vi "Create Client from Template.vi"(8 "error in (no error)":errorcluster, 9 "Generated Server Name":string="Generated Server", 10 "Target Project Path":path, 11 "Application ref in":refnum<vi>) -> (0 "error out":errorcluster, 1 "Already exists ?":bool, 2 "Server class out":refnum<vi>, 3 "Server library out":refnum<vi>)   [LabVIEW 2019, in "gRPC Scripting Tools.lvlib"]
uses:
  gRPC Scripting Tools.lvlib
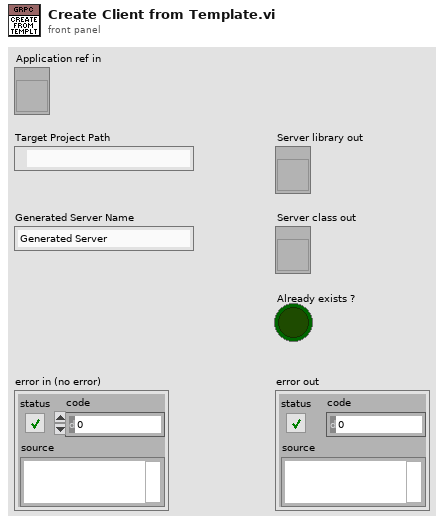
[diagram p1: front panel]
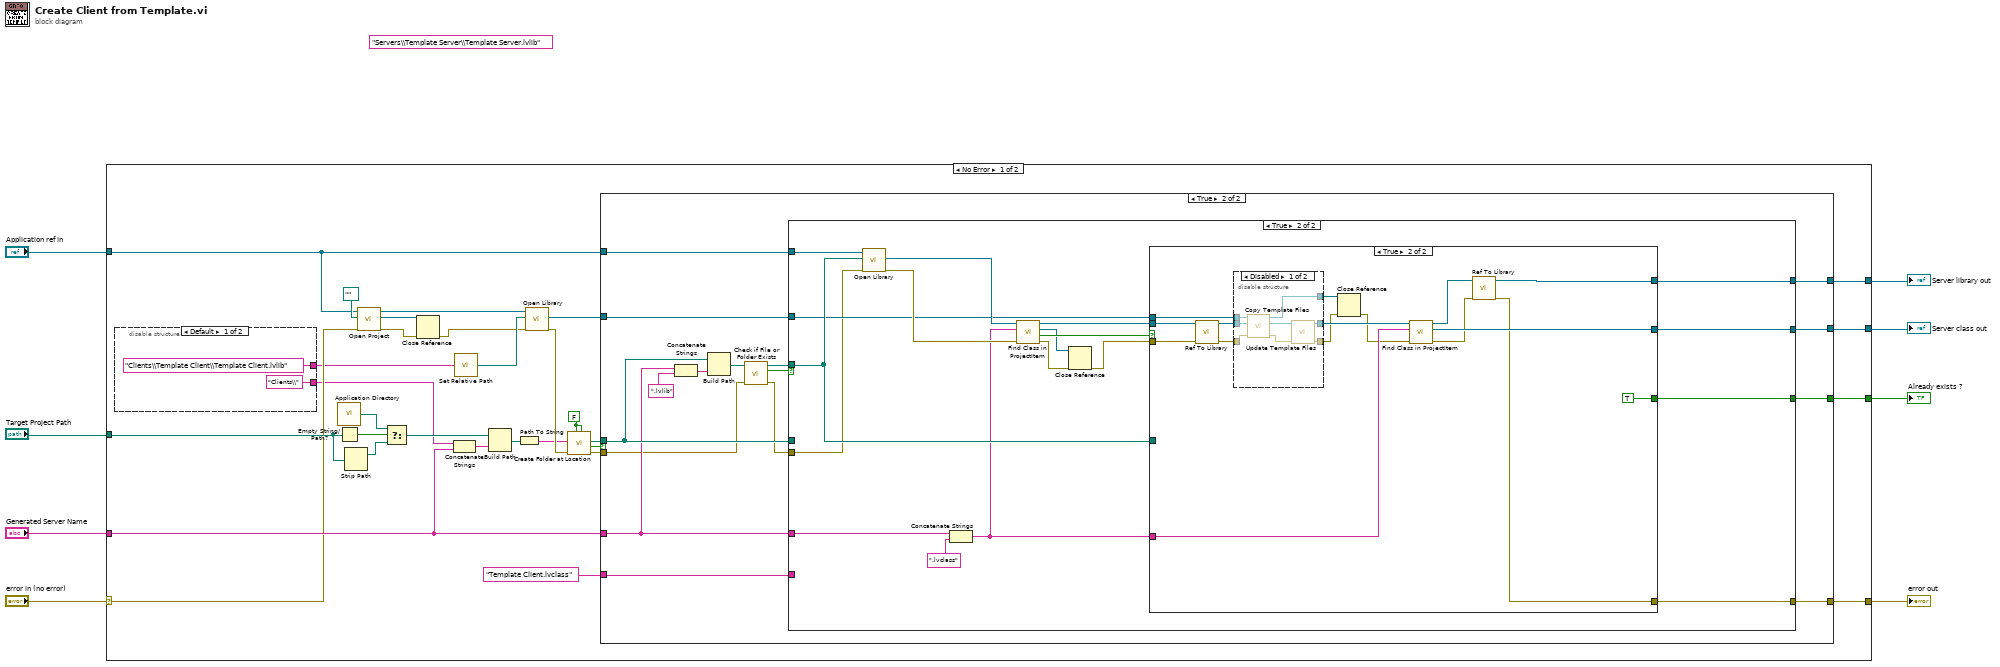
[diagram p0: block diagram]
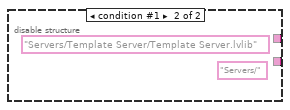
[diagram p2: hidden frame]
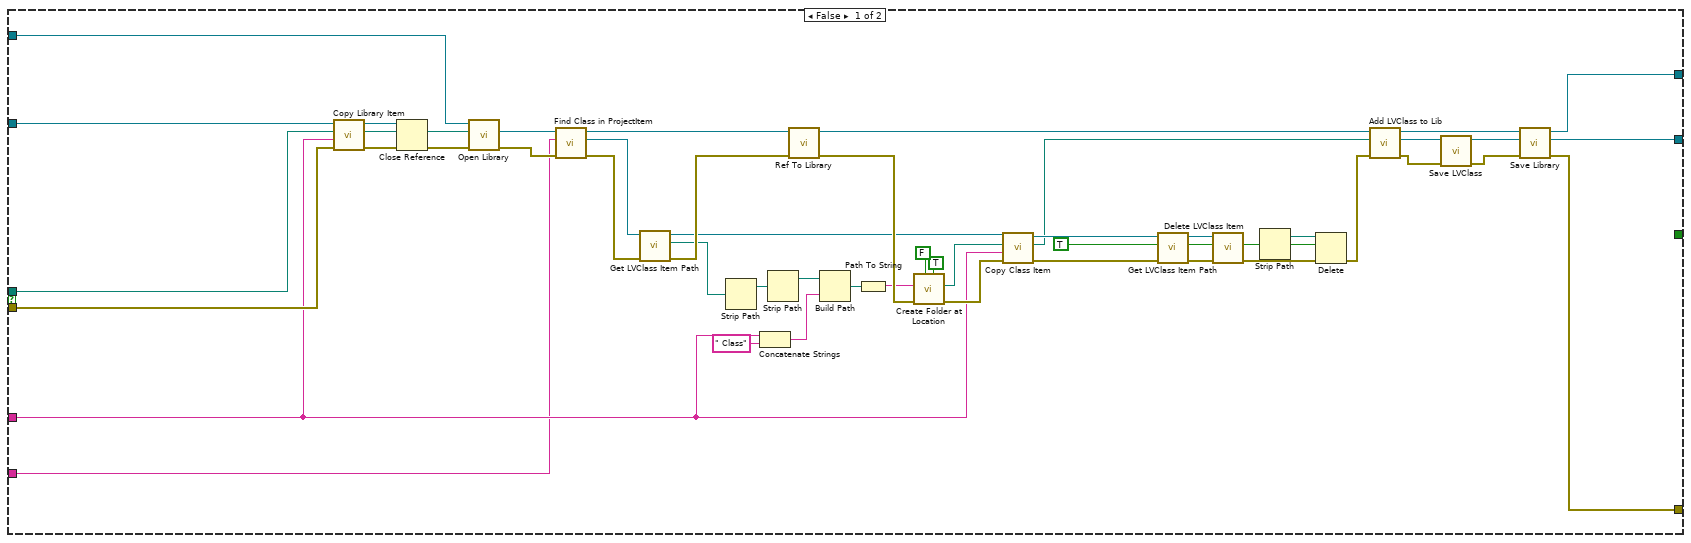
[diagram p3: hidden frame]
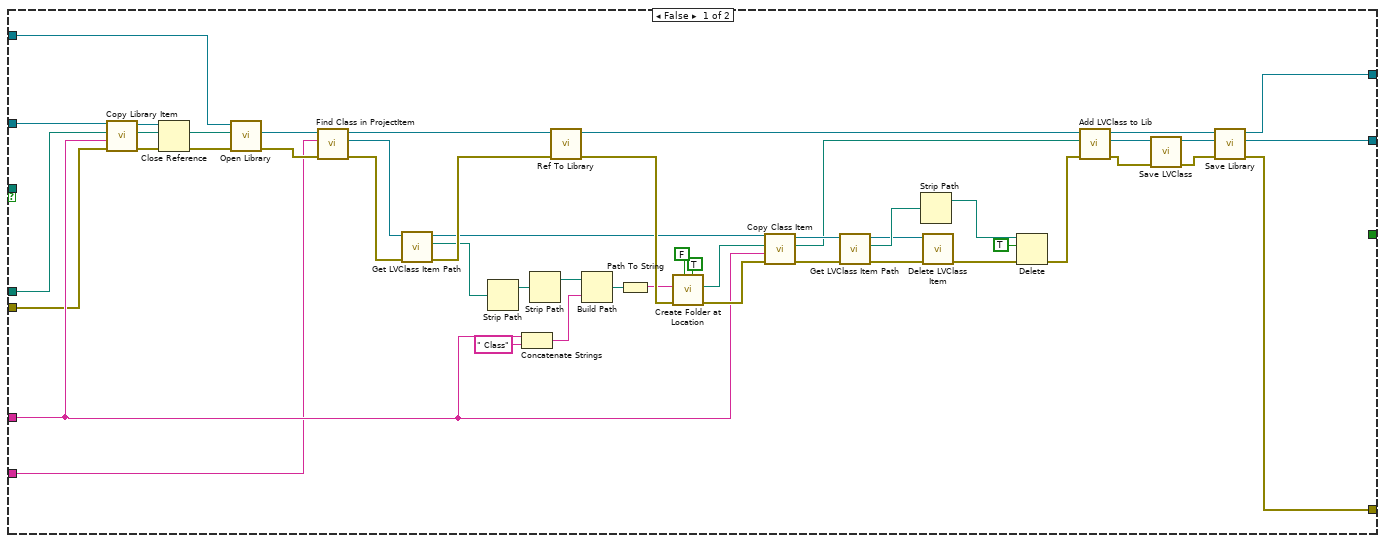
[diagram p4: hidden frame]
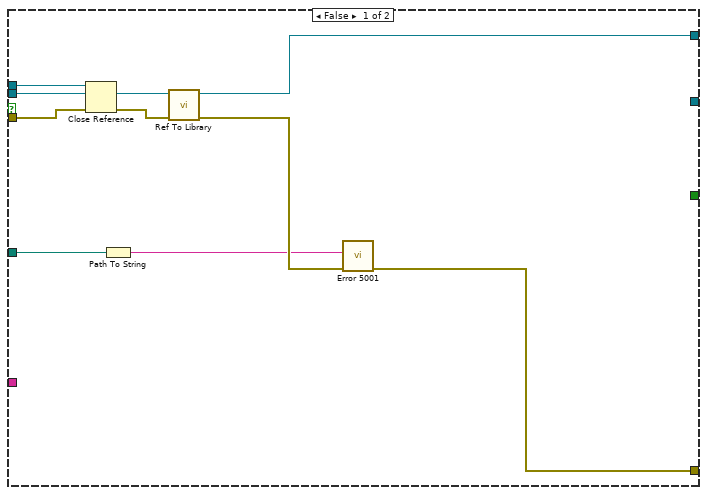
[diagram p5: hidden frame]
diagram:
  (unwired) "Servers\\Template Server\\Template Server.lvlib" ("Application Relative Path")
  n1 = case shown="No Error" "error in (no error)" {
    selector: "error in (no error)" -> [w14 w205]
    tunnel: [w38 w205] -> w8
    tunnel: [w37 _] -> w7
    tunnel: [w36 _] -> w6
    tunnel: "Target Project Path" -> [w17 _]
    tunnel: "Generated Server Name" -> [w16 _]
    tunnel: "Application ref in" -> [w15 _]
    tunnel: [w12 _] -> w1
    frame No Error {
      w29 = FALSE ("Use Relative")
      n2 = disable-structure shown="Default" {
        disable-tunnel: ["Clients\\Template Client\\Template Client.lvlib" ("Application Relative Path") _] -> w11
        disable-tunnel: ["Clients\\" ("Path") _] -> w10
        frame condition #0 (active) {
        }
        frame condition #1 {
          (unwired) "Servers/" ("Path")
          (unwired) "Servers/Template Server/Template Server.lvlib" ("Application Relative Path")
        }
      }
      n3 = call <vilib>:"Application Directory.vi"() -> ("Application Directory"=w18:path)
      n4 = Empty String/Path?(string/path=w17) -> (empty?=w21:bool)
      n5 = Strip Path(path=w17) -> (stripped path=w20:path)  [unwired: 1 out]
      n6 = call "Open Project.vi"("error in (no error)"=w14, "Project Path in"=path "", "Application reference"=w15) -> ("error out"=w24:errorcluster, "Project out"=w25:refnum<vi>, "Application out"=w32:refnum<vi>)  [unwired: 6 in]
      n7 = Select(t=w18, s=w21, f=w20) -> (s? t:f=w19:path)
      n8 = Close Reference(reference=w25, error in (no error)=w24) -> (error out=w23:errorcluster)
      n9 = Concatenate Strings(w10, w16) -> (w28:string)
      n10 = call "Set Relative Path.vi"("Application Relative Path"=w11) -> ("Full Path"=w33:path)
      n11 = Build Path(base path=w19, name or relative path=w28) -> (appended path=w27:path)
      n12 = Path To String(path=w27) -> (string=w26:string)
      n13 = call "Open Library.vi"("error in (no error)"=w23, "Full Path"=w33, "Application in"=w32) -> ("error out"=w34:errorcluster, "Library out"=w30:refnum<vi>)  [unwired: 6 in, 1 out]
      n14 = call "Create Folder at Location.vi"("Override existing (F)"=w29, "Use Relative (F)"=w29, "Error In"=w34, "Path"=w26) -> ("Error Out"=w35:errorcluster, "Already Exists ?"=w13:bool, "Full path out"=w31:path)  [unwired: 5 in]
      n15 = case shown="True" w13 {
        tunnel: [w87 w93] -> w38
        tunnel: [w86 w98] -> w37
        tunnel: [w85 w99] -> w36
        tunnel: w35 -> [w50 w90]
        tunnel: w31 -> [w49 w95]
        tunnel: w30 -> [w48 w96]
        tunnel: w16 -> [w43 w94]
        tunnel: w15 -> [w42 w97]
        tunnel: [_ w92] -> w12
        tunnel: "Template Client.lvclass" ("Class Name") -> [w41 w88]
        frame False {
          n16 = call "Copy Library Item.vi"("error in (no error)"=w50, "Copy Name"=w43, "Copy location"=w49, "Library in"=w48) -> ("error out"=w70:errorcluster, "New Lib Path"=w47:path, "Library out"=w69:refnum<vi>)  [unwired: 5 in]
          n17 = Close Reference(reference=w69, error in (no error)=w70) -> (error out=w46:errorcluster)
          n18 = call "Open Library.vi"("error in (no error)"=w46, "Full Path"=w47, "Application in"=w42) -> ("error out"=w44:errorcluster, "Library out"=w45:refnum<vi>)  [unwired: 6 in, 1 out]
          n19 = call "Find Class in ProjectItem.vi"("error in (no error)"=w44, "Class Name"=w41, "ProjectItem in"=w45) -> ("error out"=w52:errorcluster, "LVClass out"=w51:refnum<vi>, "ProjectItem out"=w64:refnum<vi>)  [unwired: 5 in, 1 out]
          n20 = call "Get LVClass Item Path.vi"("error in (no error)"=w52, "LVClassLibrary in"=w51) -> ("error out"=w66:errorcluster, "Path"=w53:path, "LVClassLibrary out"=w54:refnum<vi>)  [unwired: 7 in]
          n21 = Strip Path(path=w53) -> (stripped path=w62:path)  [unwired: 1 out]
          n22 = Concatenate Strings(w43, " Class" ("string")) -> (w57:string)
          n23 = Strip Path(path=w62) -> (stripped path=w63:path)  [unwired: 1 out]
          n24 = call "Ref To Library.vi"("error in (no error)"=w66, "ProjectItem in"=w64) -> ("error out"=w67:errorcluster, "Library out"=w80:refnum<vi>)  [unwired: 8 in]
          n25 = Build Path(base path=w63, name or relative path=w57) -> (appended path=w58:path)
          n26 = Path To String(path=w58) -> (string=w59:string)
          n27 = call "Create Folder at Location.vi"("Override existing (F)"=TRUE, "Use Relative (F)"=FALSE ("Use Relative"), "Error In"=w67, "Path"=w59) -> ("Error Out"=w68:errorcluster, "Full path out"=w61:path)  [unwired: 5 in, 1 out]
          n28 = call "Copy Class Item.vi"("error in (no error)"=w68, "New Name"=w43, "Full path in"=w61, "LVClassLibrary in"=w54) -> ("error out"=w72:errorcluster, "New Class Path out"=w65:path, "LVClassLibrary out"=w71:refnum<vi>)  [unwired: 5 in]
          n29 = call "Get LVClass Item Path.vi"("error in (no error)"=w72, "LVClassLibrary in"=w71) -> ("error out"=w74:errorcluster, "Path"=w75:path, "LVClassLibrary out"=w73:refnum<vi>)  [unwired: 7 in]
          n30 = call "Delete LVClass Item.vi"("error in (no error)"=w74, "LVClassLibrary in"=w73) -> ("error out"=w77:errorcluster)  [unwired: 9 in]
          n31 = Strip Path(path=w75) -> (stripped path=w76:path)  [unwired: 1 out]
          n32 = Delete(path (use dialog)=w76, entire hierarchy (F)=TRUE, error in=w77) -> (error out=w78:errorcluster)  [unwired: 2 in, 2 out]
          n33 = call "Add LVClass to Lib.vi"("error in (no error)"=w78, "LVClass Path in"=w65, "Library in"=w80) -> ("error out"=w83:errorcluster, "LVClassLibrary out"=w82:refnum<vi>, "Library out"=w81:refnum<vi>)  [unwired: 6 in]
          n34 = call "Save LVClass.vi"("error in (no error)"=w83, "LVClassLibrary in"=w82) -> ("error out"=w84:errorcluster, "LVClassLibrary out"=w86:refnum<vi>)  [unwired: 8 in]
          n35 = call "Save Library.vi"("error in (no error)"=w84, "Library in"=w81) -> ("error out"=w87:errorcluster, "Library out"=w85:refnum<vi>)  [unwired: 8 in]
        }
        frame True {
          n36 = Concatenate Strings(w94, ".lvlib" ("string")) -> (w102:string)
          n37 = Build Path(base path=w95, name or relative path=w102) -> (appended path=w101:path)
          n38 = call <vilib>:"Check if File or Folder Exists.vi"("error in (no error)"=w90, "path"=w101) -> ("error out"=w89:errorcluster, "file or folder exists?"=w100:bool, "dup path"=w91:path)  [unwired: 7 in]
          n39 = case shown="True" w100 {
            tunnel: [w112 w162] -> w99
            tunnel: [w111 w151] -> w98
            tunnel: w97 -> [w110 w168]
            tunnel: w96 -> [w109 w157]
            tunnel: w95 -> [w108 _]
            tunnel: w94 -> [w107 w166]
            tunnel: w89 -> [w106 w156]
            tunnel: [w105 w161] -> w93
            tunnel: [_ w159] -> w92
            tunnel: w91 -> [_ w158]
            tunnel: w88 -> [w104 _]
            frame False {
              n40 = call "Copy Library Item.vi"("error in (no error)"=w106, "Copy Name"=w107, "Copy location"=w108, "Library in"=w109) -> ("error out"=w136:errorcluster, "New Lib Path"=w116:path, "Library out"=w135:refnum<vi>)  [unwired: 5 in]
              n41 = Close Reference(reference=w135, error in (no error)=w136) -> (error out=w115:errorcluster)
              n42 = call "Open Library.vi"("error in (no error)"=w115, "Full Path"=w116, "Application in"=w110) -> ("error out"=w113:errorcluster, "Library out"=w114:refnum<vi>)  [unwired: 6 in, 1 out]
              n43 = call "Find Class in ProjectItem.vi"("error in (no error)"=w113, "Class Name"=w104, "ProjectItem in"=w114) -> ("error out"=w118:errorcluster, "LVClass out"=w117:refnum<vi>, "ProjectItem out"=w130:refnum<vi>)  [unwired: 5 in, 1 out]
              n44 = call "Get LVClass Item Path.vi"("error in (no error)"=w118, "LVClassLibrary in"=w117) -> ("error out"=w132:errorcluster, "Path"=w119:path, "LVClassLibrary out"=w120:refnum<vi>)  [unwired: 7 in]
              n45 = Strip Path(path=w119) -> (stripped path=w128:path)  [unwired: 1 out]
              n46 = Concatenate Strings(w107, " Class" ("string")) -> (w123:string)
              n47 = Strip Path(path=w128) -> (stripped path=w129:path)  [unwired: 1 out]
              n48 = call "Ref To Library.vi"("error in (no error)"=w132, "ProjectItem in"=w130) -> ("error out"=w133:errorcluster, "Library out"=w146:refnum<vi>)  [unwired: 8 in]
              n49 = Build Path(base path=w129, name or relative path=w123) -> (appended path=w124:path)
              n50 = Path To String(path=w124) -> (string=w125:string)
              n51 = call "Create Folder at Location.vi"("Override existing (F)"=TRUE, "Use Relative (F)"=FALSE ("Use Relative"), "Error In"=w133, "Path"=w125) -> ("Error Out"=w134:errorcluster, "Full path out"=w127:path)  [unwired: 5 in, 1 out]
              n52 = call "Copy Class Item.vi"("error in (no error)"=w134, "New Name"=w107, "Full path in"=w127, "LVClassLibrary in"=w120) -> ("error out"=w138:errorcluster, "New Class Path out"=w131:path, "LVClassLibrary out"=w137:refnum<vi>)  [unwired: 5 in]
              n53 = call "Get LVClass Item Path.vi"("error in (no error)"=w138, "LVClassLibrary in"=w137) -> ("error out"=w140:errorcluster, "Path"=w141:path, "LVClassLibrary out"=w139:refnum<vi>)  [unwired: 7 in]
              n54 = Strip Path(path=w141) -> (stripped path=w142:path)  [unwired: 1 out]
              n55 = call "Delete LVClass Item.vi"("error in (no error)"=w140, "LVClassLibrary in"=w139) -> ("error out"=w143:errorcluster)  [unwired: 9 in]
              n56 = Delete(path (use dialog)=w142, entire hierarchy (F)=TRUE, error in=w143) -> (error out=w144:errorcluster)  [unwired: 2 in, 2 out]
              n57 = call "Add LVClass to Lib.vi"("error in (no error)"=w144, "LVClass Path in"=w131, "Library in"=w146) -> ("error out"=w149:errorcluster, "LVClassLibrary out"=w148:refnum<vi>, "Library out"=w147:refnum<vi>)  [unwired: 6 in]
              n58 = call "Save LVClass.vi"("error in (no error)"=w149, "LVClassLibrary in"=w148) -> ("error out"=w150:errorcluster, "LVClassLibrary out"=w111:refnum<vi>)  [unwired: 8 in]
              n59 = call "Save Library.vi"("error in (no error)"=w150, "Library in"=w147) -> ("error out"=w105:errorcluster, "Library out"=w112:refnum<vi>)  [unwired: 8 in]
            }
            frame True {
              n60 = call "Open Library.vi"("error in (no error)"=w156, "Full Path"=w158, "Application in"=w168) -> ("error out"=w164:errorcluster, "Library out"=w167:refnum<vi>)  [unwired: 6 in, 1 out]
              n61 = Concatenate Strings(w166, ".lvclass" ("Class Name")) -> (w152:string)
              n62 = call "Find Class in ProjectItem.vi"("error in (no error)"=w164, "Class Name"=w152, "ProjectItem in"=w167) -> ("error out"=w154:errorcluster, "Found?"=w160:bool, "LVClass out"=w155:refnum<vi>, "ProjectItem out"=w163:refnum<vi>)  [unwired: 5 in]
              n63 = Close Reference(reference=w155, error in (no error)=w154) -> (error out=w153:errorcluster)
              n64 = case shown="True" w160 {
                tunnel: w163 -> [w177 w188]
                tunnel: [w176 w193] -> w162
                tunnel: w153 -> [w171 w190]
                tunnel: [w174 w181] -> w161
                tunnel: w158 -> [w173 _]
                tunnel: [_ TRUE] -> w159
                tunnel: w157 -> [w172 w180]
                tunnel: w152 -> [_ w187]
                tunnel: [_ w186] -> w151
                frame False {
                  n65 = Close Reference(reference=w172, error in (no error)=w171) -> (error out=w170:errorcluster)
                  n66 = Path To String(path=w173) -> (string=w169:string)
                  n67 = call "Ref To Library.vi"("error in (no error)"=w170, "ProjectItem in"=w177) -> ("error out"=w175:errorcluster, "Library out"=w176:refnum<vi>)  [unwired: 8 in]
                  n68 = call "Error 5001.vi"("error in (no error)"=w175, "Server Class Path"=w169) -> ("error out"=w174:errorcluster)  [unwired: 9 in]
                }
                frame True {
                  n69 = call "Ref To Library.vi"("error in (no error)"=w190, "ProjectItem in"=w188) -> ("error out"=w189:errorcluster, "Library out"=w191:refnum<vi>)  [unwired: 8 in]
                  n70 = disable-structure shown="Disabled" {
                    disable-tunnel: w191 -> [w201 w203]
                    disable-tunnel: w189 -> [w200 w202]
                    disable-tunnel: [w199 w203] -> w185
                    disable-tunnel: w180 -> [w198 w204]
                    disable-tunnel: [w195 w202] -> w179
                    disable-tunnel: [w194 w204] -> w178
                    frame Disabled {
                      n71 = call "Copy Template Files.vi"("error in (no error)"=w200, "Server Library (Library Item) in"=w201, "Template Library (Library Item) in"=w198) -> ("error out"=w197:errorcluster, "Server Library (Library Item) out"=w196:refnum<vi>, "Template Library (Library Item) out"=w194:refnum<vi>)  [unwired: 6 in]
                      n72 = call "Update Template Files.vi"("error in (no error)"=w197, "Server Library (Library Item) in"=w196) -> ("error out"=w195:errorcluster, "Server Library (Library Item) out"=w199:refnum<vi>)  [unwired: 8 in]
                    }
                    frame Enabled {
                    }
                  }
                  n73 = Close Reference(reference=w178, error in (no error)=w179) -> (error out=w183:errorcluster)
                  n74 = call "Find Class in ProjectItem.vi"("error in (no error)"=w183, "Class Name"=w187, "ProjectItem in"=w185) -> ("error out"=w182:errorcluster, "LVClass out"=w186:refnum<vi>, "ProjectItem out"=w184:refnum<vi>)  [unwired: 5 in, 1 out]
                  n75 = call "Ref To Library.vi"("error in (no error)"=w182, "ProjectItem in"=w184) -> ("error out"=w181:errorcluster, "Library out"=w193:refnum<vi>)  [unwired: 8 in]
                }
              }
            }
          }
        }
      }
    }
    frame Error {
    }
  }
  "error out" <- w8
  "Server class out" <- w7
  "Server library out" <- w6
  "Already exists ?" <- w1
